vi "LaserCal-Modify Header For Current Mode.vi"(0 "Options":T1, 5 "Volts":dbl[](array[numeric]), 7 "header in":string) -> (8 "header out":string)   [LabVIEW 2015]
uses:
  Typedefs/LaserCal-Options.ctl
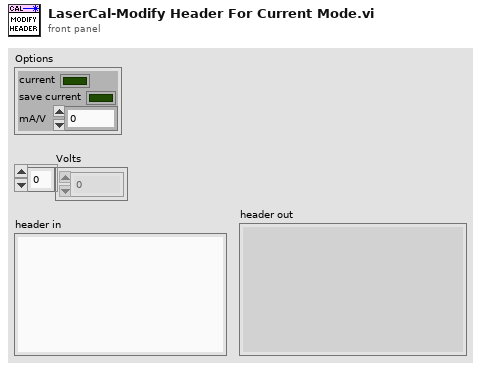
[diagram p1: front panel]
types:
  T1 = typedef "LaserCal-Options.ctl" = cluster{"current":bool, "save current":bool, "mA/V":dbl}
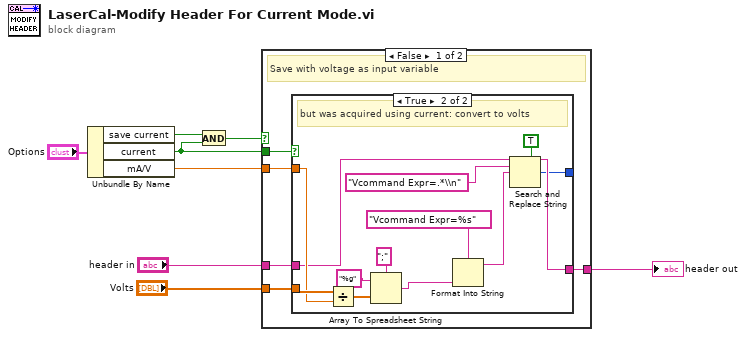
[diagram p0: block diagram]
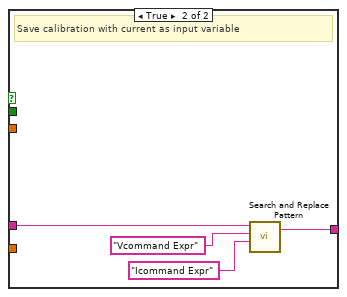
[diagram p3: hidden frame]
diagram:
  n1 = Unbundle By Name("Options") -> ("save current"=w2:bool, "current"=w6:bool, "mA/V"=w8:dbl)
  n2 = And(x=w2, y=w6) -> (x .and. y?=w3:bool)
  n3 = case shown="False" w3 {
    tunnel: "header in" -> [w13 w31]
    tunnel: [w11 w28] -> w5
    tunnel: w6 -> [w12 _]
    tunnel: "Volts" -> [w10 _]
    tunnel: w8 -> [w9 _]
    frame False {
      # "Save with voltage as input variable"
      n4 = case shown="True" w12 {
        tunnel: w13 -> [w14 w23]
        tunnel: [w14 w19] -> w11
        tunnel: w10 -> [_ w27]
        tunnel: w9 -> [_ w26]
        tunnel: [_ w17] -> _
        frame False {
          # "Normal: volts in, volts out"
        }
        frame True {
          # "but was acquired using current: convert to volts"
          n5 = Divide(x=w27, y=w26) -> (x/y=w25:dbl[])
          n6 = Array To Spreadsheet String(delimiter (Tab)=";", array=w25, 3:"%g" ("format string")) -> (spreadsheet string=w20:string)
          n7 = Format Into String(format string="Vcommand Expr=%s" ("search string"), w20) -> (resulting string=w15:string)  [unwired: 2 in, 1 out]
          n8 = Search and Replace String(multiline?=TRUE ("ignore case? (F)"), input string=w23, search string="Vcommand Expr=.*\\n", replace string=w15) -> (result string=w19:string, number of replacements=w17:i32)  [unwired: 4 in, 2 out]
        }
      }
    }
    frame True {
      # "Save calibration with current as input variable"
      n9 = call <vilib>:"Search and Replace Pattern.vi"("string"=w31, "regular expression (\"\")"="Vcommand Expr" ("regular expression (\"\")"), "replace string (\"\")"="Icommand Expr" ("regular expression (\"\")")) -> ("result string"=w28:string)  [unwired: 2 in, 1 out]
    }
  }
  "header out" <- w5
